vi "rs3_cull_faces.vi"(8 "allowed \ndepth step, mm":dbl=10.0 format="%#_13g", 10 "input vertices":dbl[][](array[numeric])=array32964x6[197784 elements], 11 "Input faces":i32[][](array[numeric])=array65200x3[195600 elements]) -> (2 "Faces  string":string[][](array[string]), 3 "output faces":i32[][](array[numeric]))   [LabVIEW 2017, in "libRealSense3.lvlib"]
uses:
  libRealSense3.lvlib
panel:
  out "depth array":dbl[](array[numeric])
  in  "Culling":T1(ring)
  out "last valid":bool
  out "last size":i32
  out "Array 3":bool[](array[boolean])=[FALSE, TRUE, FALSE, TRUE, FALSE, TRUE, FALSE, TRUE, FALSE, TRUE, FALSE, TRUE, FALSE, TRUE, FALSE, TRUE, FALSE, TRUE, FALSE, TRUE, FALSE, TRUE, FALSE, TRUE, FALSE, TRUE, FALSE, TRUE, FALSE, TRUE, FALSE, TRUE, FALSE, TRUE, FALSE, TRUE, FALSE, TRUE, FALSE, TRUE, FALSE, TRUE, FALSE, TRUE, FALSE, TRUE, FALSE, TRUE, FALSE, TRUE, FALSE, TRUE, FALSE, TRUE, FALSE, TRUE, FALSE, TRUE, FALSE, TRUE, FALSE, TRUE, FALSE, TRUE, FALSE, TRUE, FALSE, TRUE, FALSE, TRUE, FALSE, TRUE, FALSE, TRUE, FALSE, TRUE, FALSE, TRUE, FALSE, TRUE, FALSE, TRUE, FALSE, TRUE, FALSE, TRUE, FALSE, TRUE, FALSE, TRUE, FALSE, TRUE, FALSE, TRUE, FALSE, TRUE, FALSE, TRUE, FALSE, TRUE, FALSE, TRUE, FALSE, TRUE, FALSE, TRUE, FALSE, TRUE, FALSE, TRUE, FALSE, TRUE, FALSE, TRUE, FALSE, TRUE, FALSE, TRUE, FALSE, TRUE, FALSE, TRUE, FALSE, TRUE, FALSE, TRUE, FALSE, TRUE, FALSE, TRUE, FALSE, TRUE, FALSE, TRUE, FALSE, TRUE, FALSE, TRUE, FALSE, TRUE, FALSE, TRUE, FALSE, TRUE, FALSE, TRUE, FALSE, TRUE, FALSE, TRUE, FALSE, TRUE, FALSE, TRUE, FALSE, TRUE, FALSE, TRUE, FALSE, TRUE, FALSE, TRUE, FALSE, TRUE, FALSE, TRUE, FALSE, TRUE, FALSE, TRUE, FALSE, TRUE, FALSE, TRUE, FALSE, TRUE, FALSE, TRUE, FALSE, TRUE, FALSE, TRUE, FALSE, TRUE, FALSE, TRUE, FALSE, TRUE, FALSE, TRUE, FALSE, TRUE, FALSE, TRUE, FALSE, TRUE, FALSE, TRUE, FALSE, TRUE, FALSE, TRUE, FALSE, TRUE, FALSE, TRUE, FALSE, TRUE, FALSE, TRUE, FALSE, TRUE, FALSE, TRUE, FALSE, TRUE, FALSE, TRUE, FALSE, TRUE, FALSE, TRUE, FALSE, TRUE, FALSE, TRUE, FALSE, TRUE, FALSE, TRUE, FALSE, TRUE, FALSE, TRUE, FALSE, TRUE, FALSE, TRUE, FALSE, TRUE, FALSE, TRUE, FALSE, TRUE, FALSE, TRUE, FALSE, TRUE, FALSE, TRUE, FALSE, TRUE, FALSE, TRUE, FALSE, TRUE, FALSE, TRUE, FALSE, TRUE, FALSE, TRUE, FALSE, TRUE, FALSE, TRUE, FALSE, TRUE, FALSE, TRUE, FALSE, TRUE, FALSE, TRUE, FALSE, TRUE, FALSE, TRUE, FALSE, TRUE, FALSE, TRUE, FALSE, TRUE, FALSE, TRUE, FALSE, TRUE, FALSE, TRUE, FALSE, TRUE, FALSE, TRUE, FALSE, TRUE, FALSE, TRUE, FALSE, TRUE, FALSE, TRUE, FALSE, TRUE, FALSE, TRUE, FALSE, TRUE, FALSE, TRUE, FALSE, TRUE, FALSE, TRUE, FALSE, TRUE, FALSE, TRUE, FALSE, TRUE, FALSE, TRUE, FALSE, TRUE, FALSE, TRUE, FALSE, TRUE, FALSE, TRUE, FALSE, TRUE, FALSE, TRUE, FALSE, TRUE, FALSE, TRUE, FALSE, TRUE, FALSE, TRUE, FALSE, TRUE, FALSE, TRUE, FALSE, TRUE, FALSE, TRUE, FALSE, TRUE, FALSE, TRUE, FALSE, TRUE, FALSE, TRUE, FALSE, TRUE, FALSE, TRUE, FALSE, TRUE, FALSE, TRUE, FALSE, TRUE, FALSE, TRUE, FALSE, TRUE, FALSE, TRUE, FALSE, TRUE, FALSE, TRUE, FALSE, TRUE, FALSE, TRUE, FALSE, TRUE, FALSE, TRUE, FALSE, TRUE, FALSE, TRUE, FALSE, TRUE, FALSE, TRUE, FALSE, TRUE, FALSE, TRUE, FALSE, TRUE, FALSE, TRUE, FALSE, TRUE, FALSE, TRUE, FALSE, TRUE, FALSE, TRUE, FALSE, TRUE, FALSE, TRUE, FALSE, TRUE, FALSE, TRUE, FALSE, TRUE, FALSE, TRUE, FALSE, TRUE, FALSE, TRUE, FALSE, TRUE, FALSE, TRUE, FALSE, TRUE, FALSE, TRUE, FALSE, TRUE, FALSE, TRUE, FALSE, TRUE, FALSE, TRUE, FALSE, TRUE, FALSE, TRUE, FALSE, TRUE, FALSE, TRUE, FALSE, TRUE, FALSE, TRUE, FALSE, TRUE, FALSE, TRUE, FALSE, TRUE, FALSE, TRUE, FALSE, TRUE, FALSE, TRUE, FALSE, TRUE, FALSE, TRUE, FALSE, TRUE, FALSE, TRUE, FALSE, TRUE, FALSE, TRUE, FALSE, TRUE, FALSE, TRUE, FALSE, TRUE, FALSE, TRUE, FALSE, TRUE, FALSE, TRUE, FALSE, TRUE, FALSE, TRUE, FALSE, TRUE, FALSE, TRUE, FALSE, TRUE, FALSE, TRUE, FALSE, TRUE, FALSE, TRUE, FALSE, TRUE, FALSE, TRUE, FALSE, TRUE, FALSE, TRUE, FALSE, TRUE, FALSE, TRUE, FALSE, TRUE, FALSE, TRUE, FALSE, TRUE, FALSE, TRUE, FALSE, TRUE, FALSE, TRUE, FALSE, TRUE, FALSE, TRUE, FALSE, TRUE, FALSE, TRUE, FALSE, TRUE, FALSE, TRUE, FALSE, TRUE, FALSE, TRUE, FALSE, TRUE, FALSE, TRUE, FALSE, TRUE, FALSE, TRUE, FALSE, TRUE, FALSE, TRUE, FALSE, TRUE, FALSE, TRUE, FALSE, TRUE, FALSE, TRUE, FALSE, TRUE, FALSE, TRUE, FALSE, TRUE, FALSE, TRUE, FALSE, TRUE, FALSE, TRUE, FALSE, TRUE, FALSE, TRUE, FALSE, TRUE, FALSE, TRUE, FALSE, TRUE, FALSE, TRUE, FALSE, TRUE, FALSE, TRUE, FALSE, TRUE, FALSE, TRUE, FALSE, TRUE, FALSE, TRUE, FALSE, TRUE, FALSE, TRUE, FALSE, TRUE, FALSE, TRUE, FALSE, TRUE, FALSE, TRUE, FALSE, TRUE, FALSE, TRUE, FALSE, TRUE, FALSE, TRUE, FALSE, TRUE, FALSE, TRUE, FALSE, TRUE, FALSE, TRUE, FALSE, TRUE, FALSE, TRUE, FALSE, TRUE, FALSE, TRUE, FALSE, TRUE, FALSE, TRUE, FALSE, TRUE, FALSE, TRUE, FALSE, TRUE, FALSE, TRUE, FALSE, TRUE, FALSE, TRUE, FALSE, TRUE, FALSE, TRUE, FALSE, TRUE, FALSE, TRUE, FALSE, TRUE, FALSE, TRUE, FALSE, TRUE, FALSE, TRUE, FALSE, TRUE, FALSE, TRUE, FALSE, TRUE, FALSE, TRUE, FALSE, TRUE, FALSE, TRUE, FALSE, TRUE, FALSE, TRUE, FALSE, TRUE, FALSE, TRUE, FALSE, TRUE, FALSE, TRUE, FALSE, TRUE, FALSE, TRUE, FALSE, TRUE, FALSE, TRUE, FALSE, TRUE, FALSE, TRUE, FALSE, TRUE, FALSE, TRUE, FALSE, TRUE, FALSE, TRUE, FALSE, TRUE, FALSE, TRUE, FALSE, TRUE, FALSE, TRUE, FALSE, TRUE, FALSE, TRUE, FALSE, TRUE, FALSE, TRUE, FALSE, TRUE, FALSE, TRUE, FALSE, TRUE, FALSE, TRUE, FALSE, TRUE, FALSE, TRUE, FALSE, TRUE, FALSE, TRUE, FALSE, TRUE, FALSE, TRUE, FALSE, TRUE, FALSE, TRUE, FALSE, TRUE, FALSE, TRUE, FALSE, TRUE, FALSE, TRUE, FALSE, TRUE, FALSE, TRUE, FALSE, TRUE, FALSE, TRUE, FALSE, TRUE, FALSE, TRUE, FALSE, TRUE, FALSE, TRUE, FALSE, TRUE, FALSE, TRUE, FALSE, TRUE, FALSE, TRUE, FALSE, TRUE, FALSE, TRUE, FALSE, TRUE, FALSE, TRUE, FALSE, TRUE, FALSE, TRUE, FALSE]
  out "Array 2":i32[](array[numeric])=[33, 129, 32, 129, 32, 129, 33, 128, 34, 127, 34, 127, 35, 126, 35, 126, 34, 127, 36, 125, 36, 125, 37, 124, 37, 124, 36, 125, 33, 128, 33, 128, 33, 128, 33, 128, 33, 128, 33, 128, 33, 128, 33, 128, 33, 128, 34, 127, 35, 126, 36, 125, 36, 125, 35, 126, 34, 127, 34, 127, 33, 128, 33, 128, 33, 128, 33, 128, 33, 128, 33, 128, 32, 129, 32, 129, 32, 129, 32, 129, 32, 129, 32, 129, 31, 130, 32, 129, 33, 128, 33, 128, 33, 128, 33, 128, 32, 129, 32, 129, 32, 129, 32, 129, 31, 130, 31, 130, 31, 130, 31, 130, 31, 130, 31, 130, 31, 130, 32, 129, 31, 130, 30, 131, 30, 131, 31, 130, 30, 131, 31, 130, 31, 130, 31, 130, 31, 130, 31, 130, 31, 130, 32, 129, 33, 128, 34, 127, 34, 127, 34, 127, 33, 128, 32, 129, 32, 129, 32, 129, 32, 129, 31, 130, 31, 130, 31, 130, 31, 130, 31, 130, 31, 130, 31, 130, 32, 129, 33, 128, 34, 127, 34, 127, 34, 127, 34, 127, 34, 127, 33, 128, 33, 128, 32, 129, 32, 129, 33, 128, 32, 129, 33, 128, 33, 128, 33, 128, 32, 129, 31, 130, 32, 129, 32, 129, 33, 128, 33, 128, 33, 128, 33, 128, 32, 129, 32, 129, 32, 129, 31, 130, 31, 130, 30, 131, 29, 132, 30, 131, 30, 131, 30, 131, 30, 131, 30, 131, 31, 130, 31, 130, 32, 129, 32, 129, 32, 129, 31, 130, 30, 131, 30, 131, 30, 131, 30, 131, 29, 132, 29, 132, 28, 133, 28, 133, 29, 132, 29, 132, 29, 132, 30, 131, 30, 131, 30, 131, 30, 131, 31, 130, 31, 130, 31, 130, 33, 128, 33, 128, 32, 129, 31, 130, 30, 131, 30, 131, 30, 131, 31, 130, 30, 131, 30, 131, 30, 131, 30, 131, 29, 132, 29, 132, 30, 131, 30, 131, 30, 131, 30, 131, 30, 131, 30, 131, 30, 131, 31, 130, 30, 131, 29, 132, 29, 132, 29, 132, 30, 131, 30, 131, 30, 131, 30, 131, 30, 131, 30, 131, 30, 131, 31, 130, 32, 129, 32, 129, 32, 129, 32, 129, 32, 129, 33, 128, 33, 128, 32, 129, 31, 130, 31, 130, 31, 130, 30, 131, 30, 131, 31, 130, 31, 130, 30, 131, 29, 132, 29, 132, 32, 129, 32, 129, 32, 129, 33, 128, 34, 127, 34, 127, 35, 126, 35, 126, 35, 126, 36, 125, 36, 125, 37, 124, 37, 124, 37, 124, 34, 127, 33, 128, 33, 128, 33, 128, 33, 128, 33, 128, 33, 128, 33, 128, 33, 128, 34, 127, 35, 126, 36, 125, 36, 125, 36, 125, 35, 126, 34, 127, 34, 127, 33, 128, 33, 128, 33, 128, 33, 128, 33, 128, 33, 128, 32, 129, 32, 129, 32, 129, 32, 129, 32, 129, 32, 129, 32, 129, 33, 128, 33, 128, 33, 128, 33, 128, 33, 128, 32, 129, 32, 129, 32, 129, 32, 129, 31, 130, 31, 130, 31, 130, 31, 130, 31, 130, 31, 130, 32, 129, 32, 129, 31, 130, 30, 131, 31, 130, 31, 130, 31, 130, 31, 130, 31, 130, 31, 130, 31, 130, 31, 130, 32, 129, 33, 128, 34, 127, 34, 127, 34, 127, 34, 127, 32, 129, 32, 129, 32, 129, 32, 129, 32, 129, 31, 130, 31, 130, 31, 130, 31, 130, 31, 130, 31, 130, 32, 129, 33, 128, 34, 127, 34, 127, 34, 127, 34, 127, 34, 127, 34, 127, 33, 128, 33, 128, 32, 129, 33, 128, 33, 128, 33, 128, 33, 128, 33, 128, 33, 128, 32, 129, 32, 129, 32, 129, 33, 128, 33, 128, 33, 128, 33, 128, 33, 128, 32, 129, 32, 129, 32, 129, 31, 130, 31, 130, 30, 131, 30, 131, 30, 131, 30, 131, 30, 131, 30, 131, 31, 130, 31, 130, 32, 129, 32, 129, 32, 129, 32, 129, 31, 130, 30, 131, 30, 131, 30, 131, 30, 131, 29, 132, 29, 132, 28, 133, 29, 132, 29, 132, 29, 132, 30, 131, 30, 131, 30, 131, 30, 131, 31, 130, 31, 130, 31, 130, 33, 128, 33, 128, 33, 128, 31, 130, 31, 130, 30, 131, 30, 131, 31, 130, 31, 130, 30, 131, 30, 131, 30, 131, 30, 131, 29, 132, 30, 131, 30, 131, 30, 131, 30, 131, 30, 131, 30, 131, 30, 131, 31, 130, 31, 130, 29, 132, 29, 132, 29, 132, 30, 131, 30, 131, 30, 131, 30, 131, 30, 131, 30, 131, 30, 131, 31, 130, 32, 129, 32, 129, 32, 129, 32, 129, 32, 129, 33, 128, 33, 128, 33, 128, 32, 129, 31, 130, 31, 130, 31, 130, 30, 131, 31, 130, 31, 130, 31, 130, 30, 131, 29]
  out "Good faces":bool[](array[boolean])
  out "size(s)":i32[](array[numeric])=[32964, 6]
  out "Numeric":i32=65199
  out "Array":bool[](array[boolean])
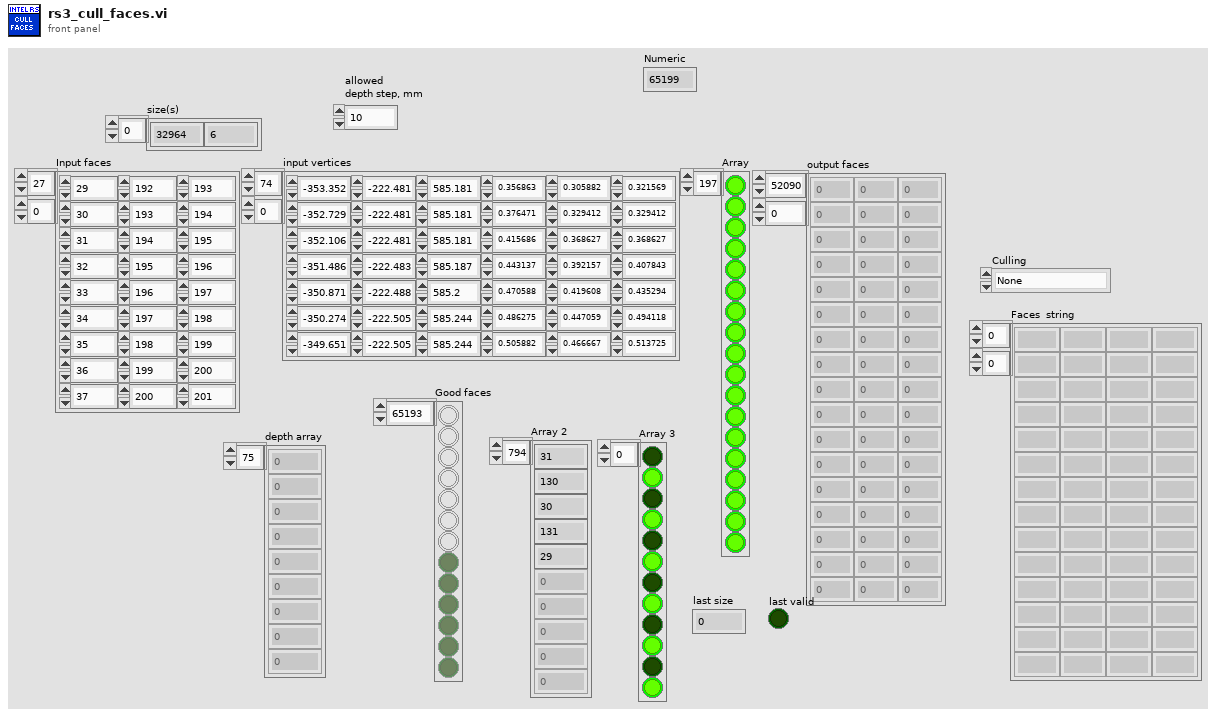
[diagram p1: front panel]
types:
  T1 = enum16{"None", "Remove faces", "Face culling", "Point culling", "Both face and point"}
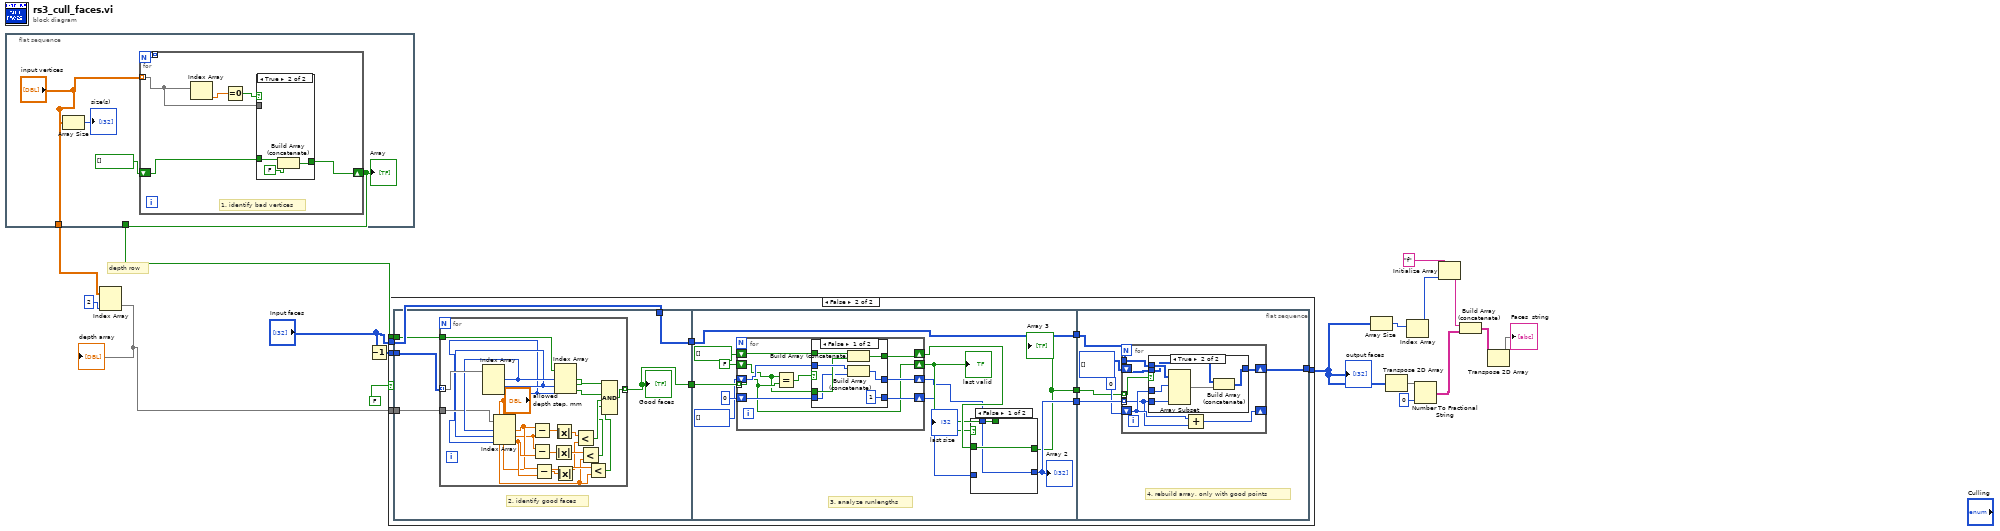
[diagram p0: block diagram]
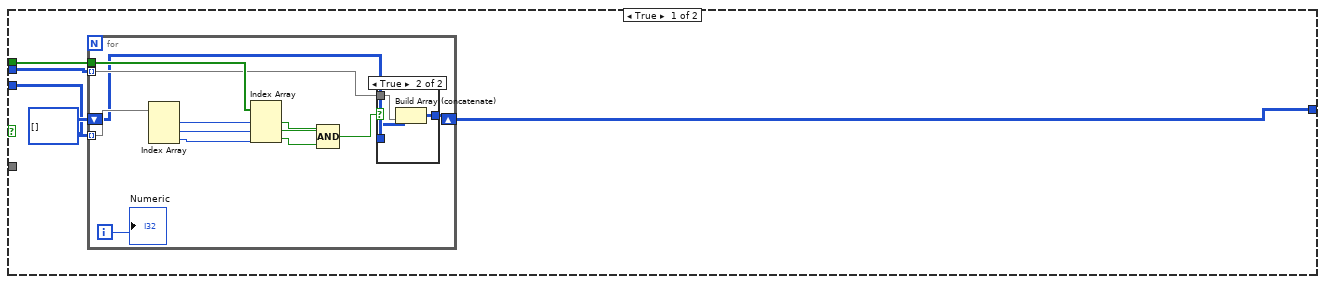
[diagram p2: hidden frame]
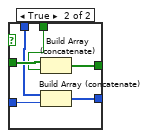
[diagram p4: hidden frame]
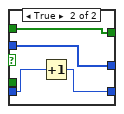
[diagram p5: hidden frame]
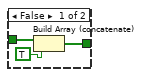
[diagram p7: hidden frame]
diagram:
  # "depth row"
  n1 = flat-sequence {
    tunnel: [w20] -> w17
    tunnel: ["input vertices"] -> w2
    frame #0 {
      n2 = Array Size(array="input vertices") -> (size(s)=→"size(s)":i32[])
      n3 = for {
        N -> [w24]
        tunnel: "input vertices" -> [w27] mode=indexing
        tunnel: [w24] -> _ mode=indexing
        shift-right: [w22] -> w20
        shift-left: bool[] [] -> [w23]
        # "1. identify bad vertices"
        n4 = Index Array(array=w27) -> (element=w25:dbl)  [unwired: 1 in]
        n5 = Equal To 0?(x=w25) -> (x = 0?=w26:bool)
        n6 = case shown="True" w26 {
          tunnel: w27 -> [_ _]
          tunnel: [w30 w31] -> w22
          tunnel: w23 -> [w28 w33]
          frame False {
            n7 = Build Array (concatenate)(w28, TRUE) -> (w30:bool[])
          }
          frame True {
            n8 = Build Array (concatenate)(w33, FALSE) -> (w31:bool[])
          }
        }
      }
      "Array" <- w20
    }
  }
  n9 = Index Array(array=w2, index (col)=2 ("index (row)")) -> (element=w1:dbl[])  [unwired: 1 in]
  "depth array" <- w1
  n10 = Decrement(x="Input faces") -> (x-1=w16:i32[][])
  n11 = case shown="False" FALSE ("Boolean") {
    tunnel: w17 -> [w38 w65]
    tunnel: w16 -> [w36 w64]
    tunnel: "Input faces" -> [w35 w62]
    tunnel: [w34 w57] -> w10
    tunnel: w1 -> [_ w56]
    frame True {
      n12 = for {
        tunnel: w36 -> [w51] mode=indexing
        tunnel: w38 -> [w47]
        tunnel: w35 -> [w42] mode=indexing
        shift-right: [w41] -> w34
        shift-left: i32[][] [] -> [w40]
        i -> [w39]
        n13 = Index Array(array=w51) -> (element #1=w50:i32, element #2=w49:i32, element #3=w48:i32)  [unwired: 3 in]
        n14 = Index Array(array=w47, index #1=w50, index #2=w49, index #3=w48) -> (element #1=w46:bool, element #2=w45:bool, element #3=w44:bool)
        n15 = Compound Arithmetic op=AND(w46, w45, w44) -> (w43:bool)
        n16 = case shown="True" w43 {
          tunnel: w42 -> [_ w55]
          tunnel: [w52 w54] -> w41
          tunnel: w40 -> [w52 w53]
          frame False {
          }
          frame True {
            n17 = Build Array (concatenate)(w53, w55) -> (w54:i32[][])
          }
        }
        "Numeric" <- w39
      }
    }
    frame False {
      n18 = flat-sequence {
        tunnel: w65 -> [w70]
        tunnel: w64 -> [w69]
        tunnel: [w68] -> w63
        tunnel: w62 -> [w68]
        tunnel: [w67] -> w61
        tunnel: w56 -> [w66]
        tunnel: w63 -> [w102]
        tunnel: w61 -> [w105]
        tunnel: [w102] -> w60
        tunnel: [w94] -> w59
        tunnel: [w95] -> w58
        tunnel: w60 -> [w139]
        tunnel: w59 -> [w136]
        tunnel: w58 -> [w138]
        tunnel: [w134] -> w57
        frame #0 {
          # "2. identify good faces"
          n19 = for {
            tunnel: w69 -> [w93] mode=indexing
            tunnel: w70 -> [w92]
            tunnel: [w88] -> w67 mode=indexing
            tunnel: w66 -> [w77]
            n20 = Index Array(array=w93) -> (element #1=w78:i32, element #2=w76:i32, element #3=w75:i32)  [unwired: 3 in]
            n21 = Index Array(array=w77, index #1=w78, index #2=w76, index #3=w75) -> (element #1=w80:dbl, element #2=w79:dbl, element #3=w81:dbl)
            n22 = Subtract(x=w80, y=w79) -> (x-y=w86:dbl)
            n23 = Subtract(x=w79, y=w81) -> (x-y=w82:dbl)
            n24 = Subtract(x=w80, y=w81) -> (x-y=w83:dbl)
            n25 = Absolute Value(x=w82) -> (abs(x)=w84:dbl)
            n26 = Absolute Value(x=w86) -> (abs(x)=w87:dbl)
            n27 = Absolute Value(x=w83) -> (abs(x)=w85:dbl)
            n28 = Index Array(array=w92, index #1=w78, index #2=w76, index #3=w75) -> (element #1=w91:bool, element #2=w90:bool, element #3=w89:bool)
            n29 = Less?(x=w87, y="allowed \ndepth step, mm") -> (x < y?=w73:bool)
            n30 = Less?(x=w84, y="allowed \ndepth step, mm") -> (x < y?=w72:bool)
            n31 = Less?(x=w85, y="allowed \ndepth step, mm") -> (x < y?=w71:bool)
            n32 = Compound Arithmetic op=AND(w91, w90, w89, w73, w72, w71) -> (w88:bool)
          }
          "Good faces" <- w67
        }
        frame #1 {
          # "3. analyze runlengths"
          n33 = for {
            tunnel: w105 -> [w117] mode=indexing
            shift-right: [w117] -> w98
            shift-left: FALSE -> [w114]
            shift-right: [w121] -> w96
            shift-left: 0 -> [w122]
            shift-right: [w120] -> w97
            shift-left: i32[] [] -> [w119]
            shift-right: [w115] -> w99
            shift-left: bool[] [] -> [w116]
            n34 = Equal?(x=w114, y=w117) -> (x = y?=w118:bool)
            n35 = case shown="False" w118 {
              tunnel: w122 -> [w123 w133]
              tunnel: [1 w132] -> w121
              tunnel: [w128 w131] -> w120
              tunnel: w119 -> [w127 w131]
              tunnel: w116 -> [w126 w130]
              tunnel: [w125 w130] -> w115
              tunnel: w114 -> [w124 _]
              frame False {
                n36 = Build Array (concatenate)(w126, w124) -> (w125:bool[])
                n37 = Build Array (concatenate)(w127, w123) -> (w128:i32[])
              }
              frame True {
                n38 = Increment(x=w133) -> (x+1=w132:i32)
              }
            }
          }
          "last size" <- w96
          "last valid" <- w98
          n39 = case shown="False" w98 {
            tunnel: w99 -> [w107 w113]
            tunnel: w98 -> [_ w112]
            tunnel: w97 -> [w106 w111]
            tunnel: w96 -> [_ w110]
            tunnel: [w106 w109] -> w95
            tunnel: [w107 w108] -> w94
            frame False {
            }
            frame True {
              n40 = Build Array (concatenate)(w113, w112) -> (w108:bool[])
              n41 = Build Array (concatenate)(w111, w110) -> (w109:i32[])
            }
          }
          "Array 3" <- w94
          "Array 2" <- w95
        }
        frame #2 {
          # "4. rebuild array, only with good points"
          n42 = for {
            shift-right: [w144] -> _
            shift-left: 0 -> [w145]
            tunnel: w139 -> [w146]
            tunnel: w138 -> [w143] mode=indexing
            shift-right: [w140] -> w134
            shift-left: i32[][] [] ("all faces input") -> [w142]
            tunnel: w136 -> [w141] mode=indexing
            n43 = case shown="True" w141 {
              tunnel: w146 -> [_ w153]
              tunnel: w145 -> [_ w152]
              tunnel: w143 -> [_ w150]
              tunnel: w142 -> [w147 w148]
              tunnel: [w147 w149] -> w140
              frame False {
              }
              frame True {
                n44 = Array Subset(array=w153, index (row)=w152, length (row)=w150) -> (w151:i32[][])  [unwired: 2 in]
                n45 = Build Array (concatenate)(w148, w151) -> (w149:i32[][])
              }
            }
            n46 = Add(x=w145, y=w143) -> (x+y=w144:i32)
          }
        }
      }
    }
  }
  "output faces" <- w10
  n47 = Array Size(array=w10) -> (size(s)=w12:i32[])
  n48 = Transpose 2D Array(2D array=w10) -> (transposed array=w9:i32[][])
  n49 = Index Array(array=w12) -> (element=w11:i32)  [unwired: 1 in]
  n50 = Number To Fractional String(number=w9, precision (6)=i16 0) -> (F-format string=w6:string[][])  [unwired: 2 in]
  n51 = Initialize Array("f", w11) -> (w7:string[])
  n52 = Build Array (concatenate)(w7, w6) -> (w5:string[][])
  n53 = Transpose 2D Array(2D array=w5) -> (transposed array=→"Faces  string":string[][])
